vi "RTM SLSC Import.vi"(8 "error in (no error)":errorcluster, 11 "Node Ptr":T1=18446744073709551615 format="%.0x") -> (0 "error out":errorcluster)   [LabVIEW 2020, in "SLSC EDS System Explorer.lvlib"]
uses:
  SLSC EDS System Explorer.lvlib
  <vilib>/NI VeriStand/Custom Device API/Custom Device Item Ref.ctl
  Shared/Constants.vi
  Shared/SLSC EDS Shared.lvlib
  SLSC CD API/SLSC CD System Explorer/SLSC CD System Explorer.lvlib
  <vilib>/NI VeriStand/Custom Device Tools/Custom Device Utility Library/Custom Device Utility Library.lvlib
  <vilib>/NI VeriStand/Custom Device API/Custom Device API.lvlib
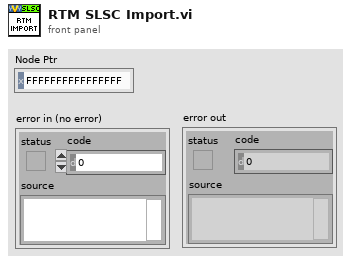
[diagram p1: front panel]
types:
  T1 = typedef "Custom Device API.lvlib/Custom Device Item Ref.ctl" = u64
  T2 = typedef "EDSjsonStructure.ctl" = cluster{"vendorNum":u32, "vendorName":string, "vendorPrefix":string, "productNum":u32, "productName":string, "capsVersion":string, "capsSpecVersion":u32, "capsSpecOldestCompatibleVersion":u32, "enums":T3[], "properties":T4[], "commands":T5[], "scales":T6[], "physicalChannels":T7[], "registerMap":cluster{"registers":T8[]}}
  T3 = typedef "enum.ctl" = cluster{"name":string, "description-en":string, "values":cluster{"name":string, "description-en":string, "value":i32}[]}
  T4 = typedef "property.ctl" = cluster{"name":string, "description-en":string, "documentation-en":string, "dataType":string, "bitfield":string, "access":string, "scale":string, "value":variant, "min":variant, "max":variant, "default value":variant}
  T5 = typedef "command.ctl" = cluster{"name":string, "description-en":string, "documentation-en":string, "startBitfield":string, "waitTimeInMs":i32, "doneBitfield":string, "doneInterrupt":string, "doneTimeoutInMs":i32, "value":variant}
  T6 = typedef "scale.ctl" = cluster{"name":string, "description-en":string, "m":dbl, "b":dbl, "forwardCoeffs":dbl[], "reverseCoeffs":dbl[], "coercion":string, "table":cluster{"scaled":dbl, "unscaled":dbl}[]}
  T7 = typedef "physicalChannel.ctl" = cluster{"name":string, "description-en":string, "commands":T5[], "properties":T4[]}
  T8 = typedef "register.ctl" = cluster{"name":string, "description-en":string, "access":string, "address":u32, "size":u32, "bitfields":cluster{"name":string, "description-en":string, "offset":u32, "size":u32, "signed":bool, "strobe":bool}[]}
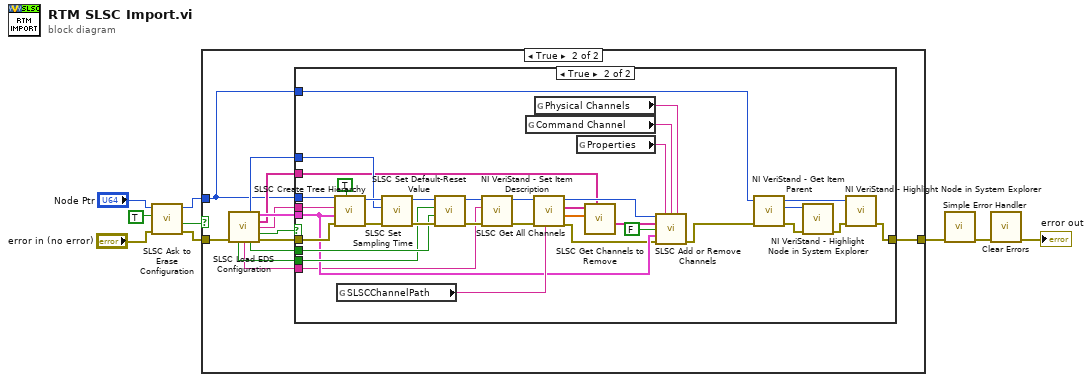
[diagram p0: block diagram]
diagram:
  n1 = call "SLSC Ask to Erase Configuration.vi"("error in (no error)"="error in (no error)", "Ask to erase?"=TRUE, "Device Item Ref in"="Node Ptr") -> ("error out"=w3:errorcluster, "Erase Data?"=w1:bool, "Item Ref out"=w2:T1)  [unwired: 5 in, 1 out]
  n2 = case shown="True" w1 {
    tunnel: [w10 w16] -> w7
    tunnel: w3 -> [w10 w12]
    tunnel: w2 -> [_ w11]
    frame False {
    }
    frame True {
      n3 = call "SLSC Load EDS Configuration.vi"("error in (no error)"=w12) -> ("Loop rate"=w21:u32, "SLSC EDS module out"=w17:T2, "Enable Channels"=w14:string[], "Custom Device Name"=w15:string, "Has capability?"=w22:bool, "Apply Default"=w19:bool, "Custom Device Description"=w13:string, "Apply Reset"=w20:bool, "error out"=w18:errorcluster)  [unwired: 5 in, 1 out]
      n4 = case shown="True" w22 {
        tunnel: w11 -> [_ w57]
        tunnel: w21 -> [_ w52]
        tunnel: w20 -> [_ w51]
        tunnel: w19 -> [_ w50]
        tunnel: w18 -> [w23 w49]
        tunnel: w17 -> [_ w40]
        tunnel: [w23 w31] -> w16
        tunnel: w15 -> [_ w37]
        tunnel: w11 -> [_ w30]
        tunnel: w14 -> [_ w29]
        tunnel: w13 -> [_ w24]
        frame False {
        }
        frame True {
          n5 = call "SLSC Create Tree Hierarchy.vi"("Initialized?"=TRUE, "error in (no error)"=w49, "SLSC EDS module"=w40, "Custom Device Name"=w37, "Item Ref in"=w57) -> ("error out"=w54:errorcluster, "Parent Ref out"=w53:T1)  [unwired: 5 in]
          n6 = global read "Constants.vi" "SLSCChannelPath"() -> (w48:string)
          n7 = call "SLSC Set Sampling Time.vi"("error in (no error)"=w54, "Loop rate"=w52, "Section Ref in"=w53) -> ("error out"=w55:errorcluster, "Channel Ref out"=w56:T1)  [unwired: 7 in]
          n8 = call "SLSC Set Default-Reset Value.vi"("error in (no error)"=w55, "Apply Reset"=w51, "Apply Default"=w50, "Section Ref in"=w56) -> ("error out"=w28:errorcluster, "Item Ref out"=w27:T1)  [unwired: 6 in]
          n9 = call <vilib>:"NI VeriStand - Set Item Description.vi"("error in (no error)"=w28, "Description"=w24, "Item Ref in"=w27) -> ("error out"=w26:errorcluster, "Item Ref out"=w25:T1)  [unwired: 7 out]
          n10 = global read "Constants.vi" "Command Channel"() -> (w44:string)
          n11 = call "SLSC Get All Channels.vi"("SLSCChannelPath"=w48, "error in (no error)"=w26, "Item Ref in"=w25) -> ("error out"=w38:errorcluster, "Channel Values"=w46:dbl[], "TreeItem Channels"=w47:string[], "Item Ref out"=w39:T1)  [unwired: 5 in]
          n12 = global read "Constants.vi" "Physical Channels"() -> (w42:string)
          n13 = global read "Constants.vi" "Properties"() -> (w43:string)
          n14 = call "SLSC Get Channels to Remove.vi"("Channels Created"=w29, "All Channel Values"=w46, "All Channels"=w47) -> ("Channels to be Deleted"=w41:string[])  [unwired: 6 in, 2 out]
          n15 = call "SLSC Add or Remove Channels.vi"("Section Ref in"=w39, "Properties"=w43, "Command Channel"=w44, "Physical Channels"=w42, "Property tree"=w41, "Add or Remove"=FALSE, "SLSC EDS module in"=w40, "error in (no error)"=w38) -> ("error out"=w32:errorcluster)  [unwired: 6 in, 1 out]
          n16 = call <vilib>:"NI VeriStand - Get Item Parent.vi"("error in (no error)"=w32, "Item Ref in"=w30) -> ("error out"=w35:errorcluster, "Parent Ref"=w33:T1, "Item Ref out"=w36:T1)  [unwired: 6 in, 1 out]
          n17 = call <vilib>:"NI VeriStand - Highlight Node in System Explorer.vi"("error in (no error)"=w35, "Item Ref in"=w33) -> ("error out"=w34:errorcluster)  [unwired: 8 in, 1 out]
          n18 = call <vilib>:"NI VeriStand - Highlight Node in System Explorer.vi"("error in (no error)"=w34, "Item Ref in"=w36) -> ("error out"=w31:errorcluster)  [unwired: 8 in, 1 out]
        }
      }
    }
  }
  n19 = call <vilib>:"Simple Error Handler.vi"("error in (no error)"=w7) -> ("error out"=w9:errorcluster)  [unwired: 4 in, 4 out]
  n20 = call <vilib>:"Clear Errors.vi"("error in (no error)"=w9) -> ("error out"=→"error out":errorcluster)  [unwired: 5 in, 1 out]
